vi "Communication - Disp PID On (eFGV).vi"(7 "Action":T1, 8 "error in":errorcluster, 11 "Disp PID in":bool[](array[boolean])) -> (0 "error out":errorcluster, 2 "Disp PID On Ref":refnum<user-event>, 3 "Disp PID out":bool[](array[boolean]))   [LabVIEW 2019]
uses:
  Controls/eFGV States.ctl
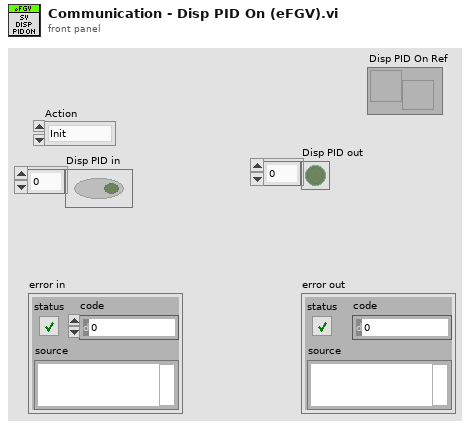
[diagram p1: front panel]
types:
  T1 = typedef "eFGV States.ctl" = enum16{"Init", "Read", "Write", "Exit"}
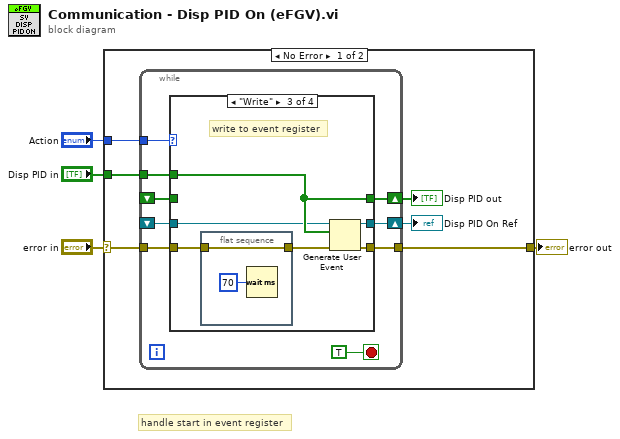
[diagram p0: block diagram]
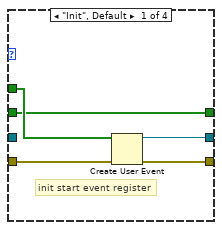
[diagram p2: hidden frame]
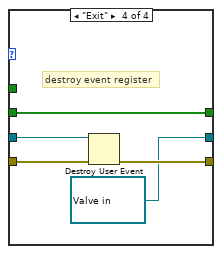
[diagram p4: hidden frame]
diagram:
  # "handle start in event register"
  n1 = case shown="No Error" "error in" {
    selector: "error in" -> [w8 w41]
    tunnel: "Action" -> [w10 _]
    tunnel: "Disp PID in" -> [w7 _]
    tunnel: [w9 w41] -> w2
    frame No Error {
      n2 = while {
        tunnel: w10 -> [w18]
        tunnel: w8 -> [w16]
        tunnel: [w15] -> w9
        shift-right: [w14] -> w6
        shift-left: _ -> [w17]
        tunnel: w7 -> [w13]
        shift-right: [w12] -> w5
        shift-left: _ -> [w11]
        stop <- TRUE stop-if-true
        n3 = case shown="\"Write\"" w18 {
          tunnel: w17 -> [w21 w26 _ w37]
          tunnel: w16 -> [w24 w27 w29 w40]
          tunnel: [w23 w27 w33 w39] -> w15
          tunnel: [w21 w26 w32 w37] -> w14
          tunnel: w13 -> [w22 _ w32 _]
          tunnel: w11 -> [_ w25 w31 w38]
          tunnel: [w20 w25 w30 refnum<user-event> refnum ("Disp PID in")] -> w12
          frame "Init", Default {
            # "init start event register"
            n4 = Create User Event(user event datatype=w22, error in=w24) -> (user event=w20:refnum<user-event>, error out=w23:errorcluster)
          }
          frame "Read" {
            # "read from event register"
          }
          frame "Write" {
            # "write to event register"
            n5 = flat-sequence {
              tunnel: [w34] -> w28
              tunnel: w29 -> [w34]
              frame #0 {
                n6 = Wait (ms)(milliseconds to wait=u32 70) -> ()  [unwired: 1 out]
              }
            }
            n7 = Generate User Event(user event=w31, event data cluster=w32, error in=w28) -> (user event out=w30:refnum<user-event>, error out=w33:errorcluster)  [unwired: 1 in]
          }
          frame "Exit" {
            # "destroy event register"
            n8 = Destroy User Event(user event=w38, error in=w40) -> (error out=w39:errorcluster)
          }
        }
      }
      "Disp PID out" <- w6
      "Disp PID On Ref" <- w5
    }
    frame Error {
    }
  }
  "error out" <- w2
